vi "OAT Output Triggered Even Angle Signal (N Channels).vi"(0 "even-angle signals":cluster{"r0":dbl, "dr":dbl, "Y":dbl[]}[](array[cluster]) {"r0" format="%.2p"; "dr" format="%.2p"; "Y" format="%.2f"}, 1 "block size":i32=-1, 2 "reset? (F)":bool, 5 "even-angle channel info":T1[](array[typedef]) {"channel info"."pregain" format="%.2f"; "channel info"."weighting filter" items=["Linear", "A-weighting", "B-weighting", "C-weighting", "ITU-R 468-4", "Dolby", "CCITT", "C-message", "Wb", "Wc", "Wd", "We", "Wf", "Wh", "Wj", "Wk", "Wm", "AES17 20 kHz lowpass", "AES17 40 kHz lowpass", "AES17 20 kHz highpass", "AES17 40 kHz highpass"]; "channel info"."dB reference" format="%^.1e"; "channel info"."engineering units" items=["custom..."=0, "V"=1, "A"=21, "C"=30, "pC"=31, "s"=32, "-"=29, "Pa"=2, "N"=20, "g"=3, "m/s^2"=4, "m/s"=5, "m"=6, "mm/s"=12, "mm"=13, "micron/s"=14, "micron"=15, "in/s^2"=7, "in/s"=8, "in"=9, "mil/s"=10, "mil"=11, "rad/s^2"=16, "rad/s"=17, "rad"=18, "deg/s^2"=26, "deg/s"=27, "deg"=28, "RPM"=22, "cycle/s^2"=23, "Hz"=24, "cycle"=25, "strain"=19]; "channel info"."sensor sensitivity" format="%#_5f"}, 11 "error in (no error)":errorcluster, 12 "trigger period [rev]":dbl=1.0) -> (4 "triggered even-angle signals":cluster{"r0":dbl, "dr":dbl, "Y":dbl[]}[](array[cluster]) {"r0" format="%.2p"; "dr" format="%.2p"; "Y" format="%.2f"}, 6 "even-angle channel info out":T1[](array[typedef]) {"channel info"."pregain" format="%.2f"; "channel info"."weighting filter" items=["Linear", "A-weighting", "B-weighting", "C-weighting", "ITU-R 468-4", "Dolby", "CCITT", "C-message", "Wb", "Wc", "Wd", "We", "Wf", "Wh", "Wj", "Wk", "Wm", "AES17 20 kHz lowpass", "AES17 40 kHz lowpass", "AES17 20 kHz highpass", "AES17 40 kHz highpass"]; "channel info"."dB reference" format="%^.1e"; "channel info"."engineering units" items=["custom..."=0, "V"=1, "A"=21, "C"=30, "pC"=31, "s"=32, "-"=29, "Pa"=2, "N"=20, "g"=3, "m/s^2"=4, "m/s"=5, "m"=6, "mm/s"=12, "mm"=13, "micron/s"=14, "micron"=15, "in/s^2"=7, "in/s"=8, "in"=9, "mil/s"=10, "mil"=11, "rad/s^2"=16, "rad/s"=17, "rad"=18, "deg/s^2"=26, "deg/s"=27, "deg"=28, "RPM"=22, "cycle/s^2"=23, "Hz"=24, "cycle"=25, "strain"=19]; "channel info"."sensor sensitivity" format="%#_5f"}, 15 "error out":errorcluster)   [LabVIEW 2017, in "SoundVib_OAUtility.lvlib"]
doc: "Generates triggered even-angle signals for vector averaging in order power spectrum calculations. Use this VI to remove uncorrelated phenomenon for vector averaging. Each instance of this VI maintains its own state; use the N Waveforms instance of this VI to process an array of channels. Wire data to the <B>even-angle signal</B> input to determine the polymorphic instance to use or manually select the instance."
uses:
  <vilib>/addons/Sound and Vibration/Order Analysis/Utility/SoundVib_OAUtility.lvlib
  <vilib>/addons/_NISVFA/_Shared subVIs/Controls/svc_Resampled Channel Info.ctl
  <vilib>/addons/_NISVFA/_Shared subVIs/Controls/svc_Channel Info.ctl
  <vilib>/addons/_NISVFA/_Shared subVIs/Controls/svc_Engineering Units Text Ring.ctl
  <vilib>/addons/_NISVFA/_Shared subVIs/Controls/svc_Weighting Filter Text Ring.ctl
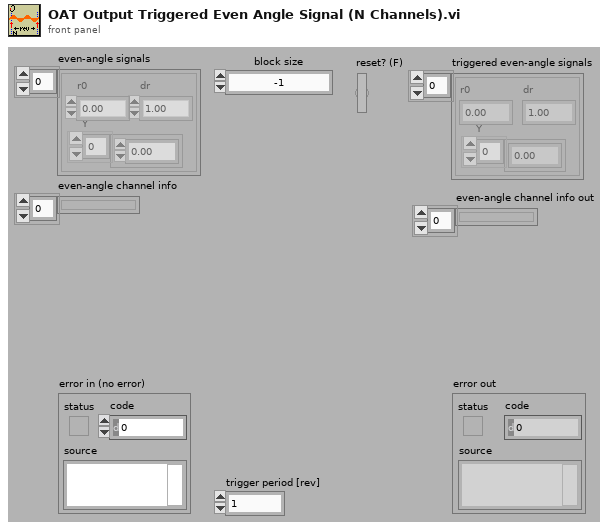
[diagram p1: front panel]
types:
  T1 = typedef "svc_Resampled Channel Info.ctl" = cluster{"channel name":string, "description":string, " channel info":T2}
  T2 = typedef "svc_Channel Info.ctl" = cluster{"sensor sensitivity":dbl, "engineering units":T3, "dB reference":dbl, "custom label":string, "weighting filter":T4, "pregain":dbl}
  T3 = typedef "svc_Engineering Units Text Ring.ctl" = u16
  T4 = typedef "svc_Weighting Filter Text Ring.ctl" = u16
  T5 = cluster{"ignore dt's equal":bool, "ignore array lengths equal":bool, "ignore # channels":bool}
  T6 = cluster{"ignore dt":bool, "ignore t0 continuity":bool, "ignore array length":bool, "ignore channel info":bool, "ignore channel name":bool}
  T7 = cluster{"r0":dbl, "dr":dbl, "even angle signal":dbl[]}[]
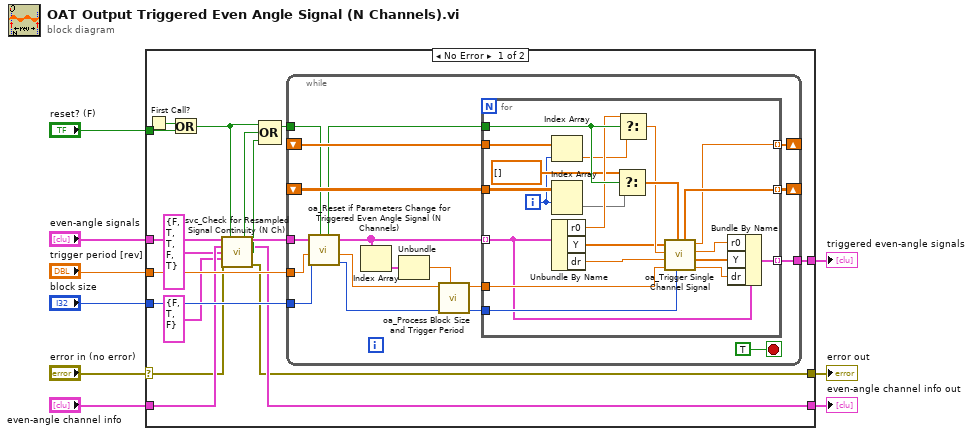
[diagram p0: block diagram]
diagram:
  n1 = case shown="No Error" "error in (no error)" {
    selector: "error in (no error)" -> [w13 w67]
    tunnel: [w12 w67] -> w8
    tunnel: "even-angle signals" -> [w25 w66]
    tunnel: "even-angle channel info" -> [w14 w65]
    tunnel: [w15 w65] -> w5
    tunnel: [w24 w66] -> w4
    tunnel: "trigger period [rev]" -> [w23 _]
    tunnel: "block size" -> [w22 _]
    tunnel: "reset? (F)" -> [w21 _]
    frame No Error {
      n2 = First Call?() -> (First Call?: T/F=w20:bool)
      n3 = Or(x=w20, y=w21) -> (x .or. y?=w17:bool)
      n4 = call <vilib>:"svc_Check for Resampled Signal Continuity (N Ch).vi"("even angle signals"=w25, "restart averaging (F)"=w17, "even angle channel info"=w14, "parameter controls"=T6 {"ignore dt"=FALSE, "ignore t0 continuity"=TRUE, "ignore array length"=TRUE, "ignore channel info"=FALSE, "ignore channel name"=TRUE}, "multichannel parameter controls"=T5 {"ignore dt's equal"=FALSE, "ignore array lengths equal"=TRUE, "ignore # channels"=FALSE}, "error in (no error)"=w13) -> ("dup even angle signals"=w19:T7, "dup even angle channel info"=w15:T1[], "waveform parameter changed"=w16:bool, "error out"=w12:errorcluster)  [unwired: 3 in, 3 out]
      n5 = Compound Arithmetic op=OR(w17, w16, w16) -> (w18:bool)
      n6 = while {
        shift-right: [w42] -> _
        shift-left: _ -> [w43]
        shift-right: [w41] -> _
        shift-left: _ -> [w38]
        tunnel: [w40] -> w24
        tunnel: w19 -> [w27]
        tunnel: w23 -> [w31]
        tunnel: w22 -> [w29]
        tunnel: w18 -> [w26]
        stop <- TRUE stop-if-true
        n7 = call <vilib>:"oa_Reset if Parameters Change for Triggered Even Angle Signal (N Channels).vi"("reset? (T)"=w26, "block size"=w29, "trigger period [rev]"=w31, "even angle signals"=w27) -> ("block size out"=w28:i32, "trigger period out [rev]"=w30:dbl, "even angle signals out"=w33:cluster{"r0":dbl, "dr":dbl, "Y":dbl[]}[], "reset out"=w32:bool)  [unwired: 4 in]
        n8 = Index Array(array=w33) -> (element=w35:cluster{"r0":dbl, "dr":dbl, "Y":dbl[]})  [unwired: 1 in]
        n9 = Unbundle(w35) -> ("dr"=w34:dbl)  [unwired: 2 out]
        n10 = call <vilib>:"oa_Process Block Size and Trigger Period.vi"("dr"=w34, "block size"=w28, "trigger period [rev]"=w30) -> ("block size out"=w36:i32, "trigger period out [rev]"=w37:dbl)  [unwired: 7 in]
        n11 = for {
          tunnel: w43 -> [w64]
          tunnel: w38 -> [w46]
          tunnel: [w59] -> w42 mode=indexing
          tunnel: [w58] -> w41 mode=indexing
          tunnel: [w57] -> w40 mode=indexing
          tunnel: w32 -> [w50]
          tunnel: w33 -> [w56] mode=indexing
          tunnel: w36 -> [w60]
          tunnel: w37 -> [w61]
          i -> [w44]
          n12 = Index Array(array=w46, index=w44) -> (element=w45:dbl)
          n13 = Index Array(array=w64, index (row)=w44) -> (element=w47:dbl[])  [unwired: 1 in]
          n14 = Unbundle By Name(w56) -> ("r0"=w49:dbl, "Y"=w52:dbl[], "dr"=w51:dbl)
          n15 = Select(t=dbl[] [] ("Y"), s=w50, f=w47) -> (s? t:f=w63:dbl[])
          n16 = Select(t=w49, s=w50, f=w45) -> (s? t:f=w62:dbl)
          n17 = call <vilib>:"oa_Trigger Single Channel Signal.vi"("block size"=w60, "history signal"=w63, "trigger period [rev]"=w61, "dr"=w51, "history r0"=w62, "signal to be triggered"=w52) -> ("dr out"=w53:dbl, "triggered signal"=w54:dbl[], "triggered r0"=w55:dbl, "history r0"=w58:dbl, "history signal out"=w59:dbl[])  [unwired: 1 in]
          n18 = Bundle By Name(cluster=w56, "r0"=w55, "Y"=w54, "dr"=w53) -> (w57:cluster{"r0":dbl, "dr":dbl, "Y":dbl[]})
        }
      }
    }
    frame Error {
    }
  }
  "error out" <- w8
  "triggered even-angle signals" <- w4
  "even-angle channel info out" <- w5
